vi "Split 1 D Array.vi"() -> ()   [LabVIEW 2015]
panel:
  in  "Tab Control":enum32{"Page 1", "Page 2"}(tab)
  out "Array":dbl[](array[numeric])
  out "first subarray":dbl[](array[numeric])
  out "second subarray":dbl[](array[numeric])
  in  "index":i32
  # "Split 1 D Array"
  # "Pardeep Kumar"
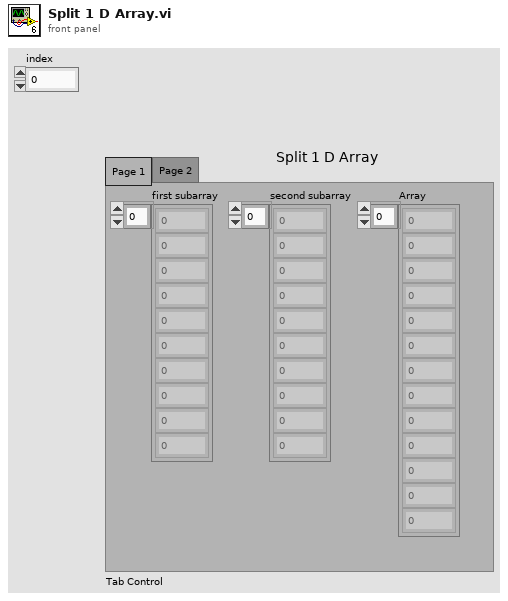
[diagram p1: front panel]
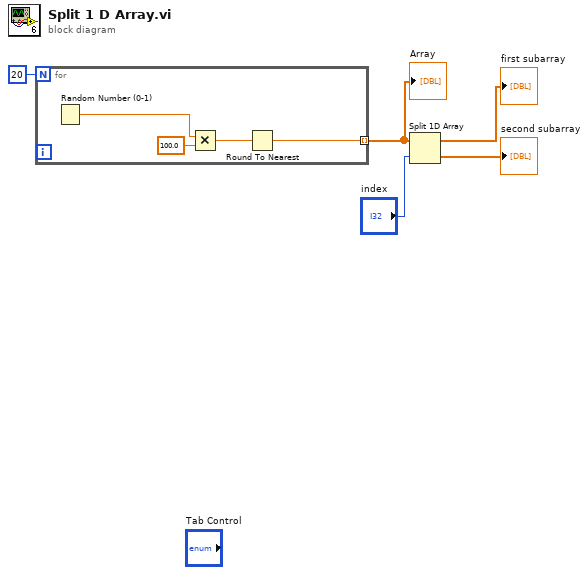
[diagram p0: block diagram]
diagram:
  n1 = for {
    N: 20 -> [_]
    tunnel: [w6] -> w5 mode=indexing
    n2 = Random Number (0-1)() -> (number: 0 to 1=w9:dbl)
    n3 = Multiply(x=w9, y=100.0) -> (x*y=w7:dbl)
    n4 = Round To Nearest(number=w7) -> (nearest integer value=w6:dbl)
  }
  "Array" <- w5
  n5 = Split 1D Array(array=w5, index="index") -> (first subarray=→"first subarray":dbl[], second subarray=→"second subarray":dbl[])
